vi "execute.vi"(8 "error in (no error)":errorcluster, 10 "Context in":refnum<class "Context.lvclass">, 11 "EnterMaintenanceCommand in":refnum<class "EnterMaintenanceCommand.lvclass">) -> (0 "error out":errorcluster, 2 "Context out":refnum<class "Context.lvclass">, 3 "EnterMaintenanceCommand out":refnum<class "EnterMaintenanceCommand.lvclass">)   [LabVIEW 2016, in "EnterMaintenanceCommand.lvclass"]
uses:
  EnterMaintenanceCommand.lvclass
  Context/Context.lvclass
  EnterMaintenanceCommand.lvclass/EnterMaintenanceCommand.ctl
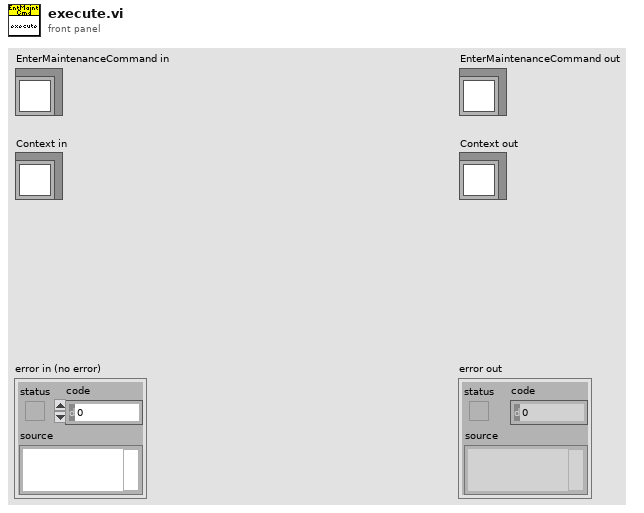
[diagram p1: front panel]
types:
  T1 = typedef "M1M3SupportTopics.lvlib/CommandEnterMaintenance.ctl" = cluster{"CommandId":T2, "EnterMaintenance":bool}
  T2 = typedef "M1M3SupportTopics.lvlib/CommandId.ctl" = i32
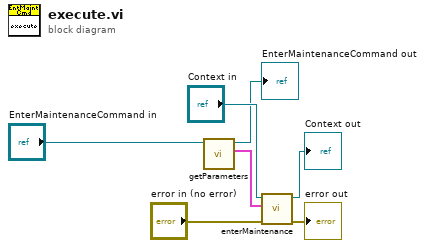
[diagram p0: block diagram]
diagram:
  n1 = call "getParameters.vi"("EnterMaintenanceCommand in"="EnterMaintenanceCommand in") -> ("Parameters"=w5:T1, "EnterMaintenanceCommand out"=→"EnterMaintenanceCommand out":refnum<class "EnterMaintenanceCommand.lvclass">)  [unwired: 9 in]
  n2 = call "enterMaintenance.vi"("error in (no error)"="error in (no error)", "Parameters"=w5, "Context in"="Context in") -> ("error out"=→"error out":errorcluster, "Context out"=→"Context out":refnum<class "Context.lvclass">)  [unwired: 7 in]
